vi "hmi_simRK4serial.vi"() -> ()   [LabVIEW 2017]
uses:
  Control 6.ctl
  <vilib>/Utility/miscctls.llb/LVBoundsTypeDef.ctl
  <vilib>/Instr/_visa.llb/VISA Configure Serial Port (Instr).vi
  <vilib>/MakerHub/LINX/LMH-LINX.lvlib
panel:
  in  "ENVIAR":bool=TRUE
  out "bomba":dbl
  out "dato a enviar":string
  in  "stop":bool
  out "time array":dbl[](array[numeric])
  in  "Tab Control":enum32{"HMI", "Monitorizacion de flujo"}(tab)
  out "Boolean 2":bool
  out "FUGA 1":bool
  out "FUGA 2":bool
  out "u2":dbl=3.4 format="%#_13g"
  out "Boolean":bool
  in  "BOMBA ON/OFF":bool
  out "FT1":bool(c317)
  in  "valvula 1":bool
  in  "valvula 2":bool
  out "TEE 02":bool
  out "TUBERIA 1IN TRAMO 02":bool(c317)
  out "TEE1":bool
  out "Multi-Segment Pipe 2":T1
  out "Multi-Segment Pipe 3":bool(c317)
  out "Multi-Segment Pipe 4":bool(c317)
  out "FT2":bool(c317)
  out "FT 1":dbl caption="L/min"
  out "FT 2":dbl caption="L/min"
  out "67.5°":bool
  out "45°":bool
  out "22.5°":bool
  out "90°":bool
  out "TANQUE\n FLUIDO:AGUA":dbl(slide) scale=0.0..100.0
  out "SENSOR FLUJO":bool
  out "67.5° 3":bool
  out "45° 3":bool
  out "22.5° 3":bool
  out "90° 3":bool
  out "SENSOR FLUJO 3":bool
  out "BOMBA 1/2 HP":bool
  out "tiempo":dbl
  in  "Flujo de entrada":dbl=0.00425 format="%#_13g"
  out "codo90":bool
  out "u1":dbl=6.0 format="%#_13g"
  in  "Tiempo muestreo":i32=200
  out "periodo":dbl
  in  "Flujo de salida":dbl=0.00425 format="%#_13g"
  out "element":dbl
  out "element 2":dbl
  in  "Puerto sensores":refnum<visa-resource-name>="COM3"
  in  "GUARDAR DATOS":bool
  out "Flujo de entrada y salida":cluster{dbl[], dbl[]}[](graph)
  out "Freq2":dbl
  out "Freq1":dbl
  out "Cluster":T2
  out "SIMULACION DE Q1 y Q2":cluster{dbl[], dbl[]}[](graph)
  out "SIMULACION DE H2":cluster{"time array":dbl[], dbl[]}(graph)
  # "PVC  1\" FLUJO: AGUA"
  # "PVC  1/2\" FLUJO: AGUA"
  # "FUGA 1"
  # "2.5 m"
  # "PVC  1/2\" FLUJO: AGUA"
  # "FUGA 2"
  # "PVC  1\" FLUJO: AGUA"
  # "6 m"
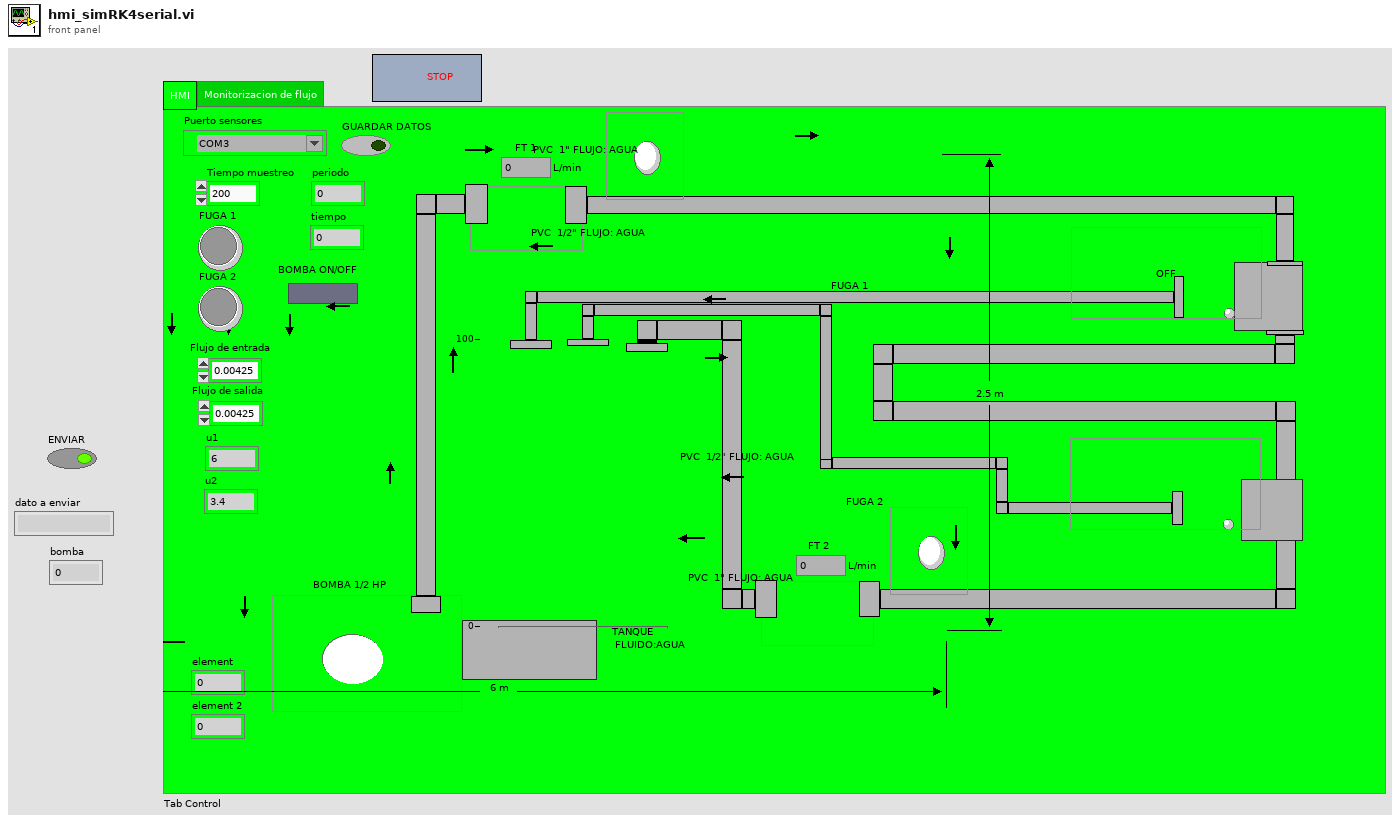
[diagram p1: front panel]
types:
  T1 = typedef "Control 6.ctl" = bool
  T2 = cluster{"FLUJO DE ENTRADA":dbl, "FLUJO DE SALIDA":dbl, "VOLUMEN 1 (L) ":dbl, "VOLUMEN 2 (L) ":dbl}
  T3 = typedef "LVBoundsTypeDef.ctl" = cluster{"Width":u32, "Height":u32}
  T4 = cluster{"index":i32, "index 2":i32, "index 3":i32, "index 4":i32, "index 5":i32, "index 6":i32, i32, i32, i32}
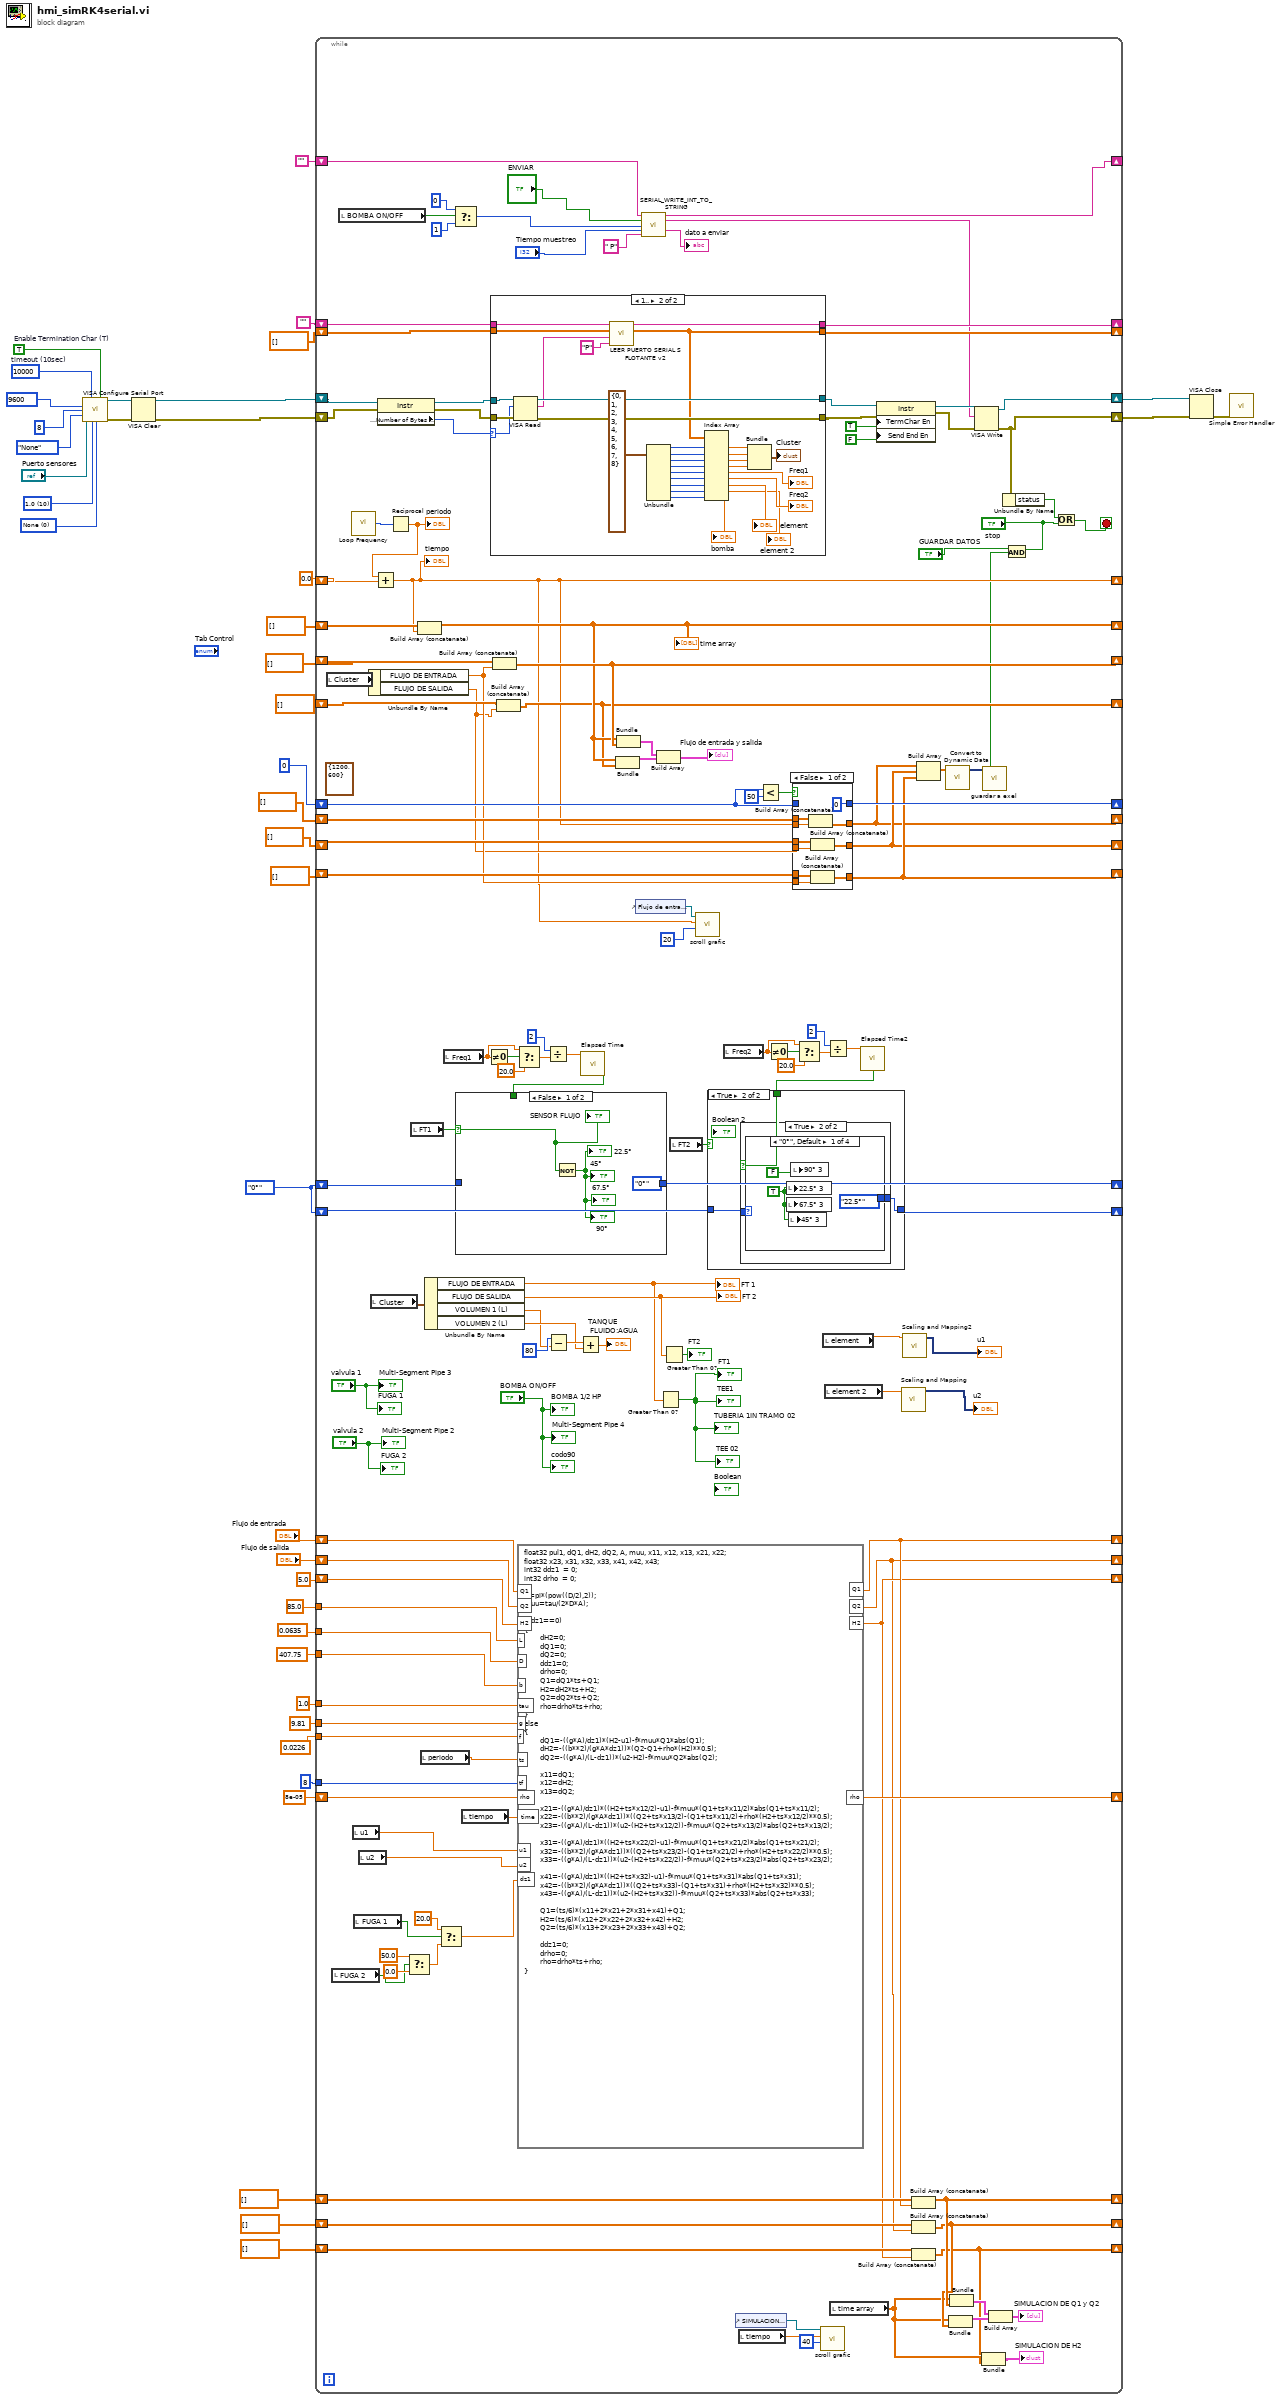
[diagram p0: block diagram]
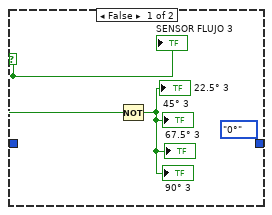
[diagram p2: hidden frame]
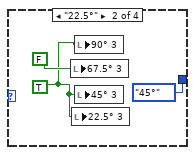
[diagram p4: hidden frame]
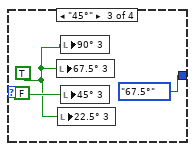
[diagram p5: hidden frame]
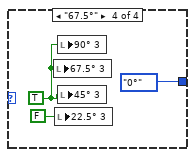
[diagram p6: hidden frame]
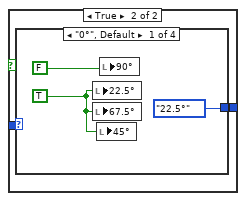
[diagram p8: hidden frame]
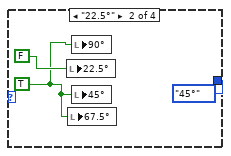
[diagram p9: hidden frame]
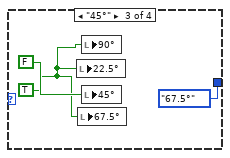
[diagram p10: hidden frame]
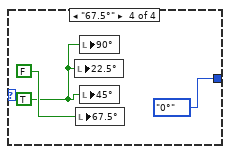
[diagram p11: hidden frame]
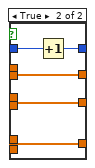
[diagram p12: hidden frame]
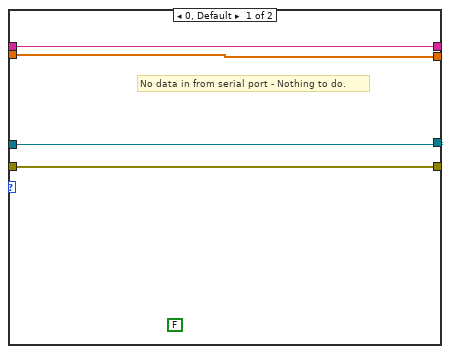
[diagram p13: hidden frame]
diagram:
  w21 = 9600 items=["9600"=9600, "19200"=19200, "38400"=38400, "57600"=57600, "74880"=74880, "115200"=115200] ("BaudRate")
  w20 = enum16{"0°", "22.5°", "45°", "67.5°"}."0°"
  w33 = u16 10 items=["1.0"=10, "1.5"=15, "2.0"=20] ("stop bits (10: 1 bit)")
  w34 = u16 0 items=["None", "XON/XOFF", "RTS/CTS", "XON/XOFF & RTS/CTS", "DTR/DSR", "XON/XOFF & DTR/DSR"] ("flow control (0:none)")
  w39 = TRUE  # Enable Termination Char (T)
  w40 = u32 10000  # timeout (10sec)
  (unwired) T3 {"Width"=1200, "Height"=600} ("Tab Control Pane Dimension")
  n1 = call-poly "VISA Configure Serial Port"("VISA resource name"="Puerto sensores", "timeout (10sec)"=w40, "Enable Termination\nChar (T)"=w39, "baud rate (9600)"=w21, "data bits (8)"=u16 8 ("Data bits (8)"), "parity (0:none)"=enum16{"None", "Odd", "Even", "Mark", "Space"}."None" ("Parity (0:none)"), "stop bits (10: 1 bit)"=w33, "flow control (0:none)"=w34) -> ("VISA resource name out"=w37:refnum<visa-resource-name>, "error out"=w38:errorcluster)  [unwired: 6 in]
  n2 = VISA Clear(VISA resource name=w37, error in (no error)=w38) -> (VISA resource name out=w36:refnum<visa-resource-name>, error out=w2:errorcluster)
  n3 = while {
    shift-right: [w155] -> _
    shift-left: dbl[] [] -> [w175]
    shift-right: [w72] -> _
    shift-left: 0.0 -> [w176]
    shift-right: [w168] -> _
    shift-left: dbl[] [] -> [w173]
    shift-right: [w154] -> _
    shift-left: dbl[] [] -> [w174]
    shift-right: [w165] -> _
    shift-left: 0 -> [w166]
    shift-right: [w160] -> _
    shift-left: dbl[] [] -> [w163]
    shift-right: [w161] -> _
    shift-left: dbl[] [] -> [w162]
    shift-right: [w159] -> _
    shift-left: dbl[] [] -> [w164]
    shift-right: [w58] -> w41
    shift-left: w2 -> [w60]
    shift-right: [w45] -> w22
    shift-left: w36 -> [w179]
    shift-right: [w140] -> _
    shift-left: w20 -> [w139]
    shift-right: [w120] -> _
    shift-left: w20 -> [w129]
    shift-right: [w116] -> _
    shift-left: "" -> [w117]
    shift-right: [w114] -> _
    shift-left: dbl[] [] -> [w115]
    tunnel: 0.0226 ("input variable") -> [w112]
    tunnel: 9.81 ("input variable") -> [w111]
    tunnel: 1.0 ("input variable") -> [w110]
    tunnel: 407.75 ("input variable") -> [w109]
    tunnel: 0.0635 ("D") -> [w108]
    tunnel: 85.0 ("L") -> [w107]
    shift-right: [w87] -> _
    shift-left: "Flujo de entrada" -> [w106]
    shift-right: [w76] -> _
    shift-left: "Flujo de salida" -> [w105]
    shift-right: [w84] -> _
    shift-left: 5.0 -> [w104]
    shift-right: [w102] -> _
    shift-left: 8e-05 -> [w103]
    tunnel: 8 -> [w101]
    shift-right: [w80] -> _
    shift-left: dbl[] [] -> [w88]
    shift-right: [w79] -> _
    shift-left: dbl[] [] -> [w86]
    shift-right: [w68] -> _
    shift-left: dbl[] [] -> [w85]
    shift-right: [w55] -> _
    shift-left: "" -> [w56]
    stop <- w113 stop-if-true
    n4 = local read "Cluster"() -> (w153:T2)
    n5 = local read "FUGA 2"() -> (w94:bool)
    n6 = local read "BOMBA ON/OFF"() -> (w50:bool)
    n7 = call <vilib>:"Loop Frequency.vi"() -> ("Loop Rate (Hz)"=w170:u32)
    n8 = local read "u1"() -> (w74:dbl)
    n9 = local read "FUGA 1"() -> (w95:bool)
    n10 = local read "u2"() -> (w73:dbl)
    n11 = Unbundle By Name(w153) -> ("FLUJO DE ENTRADA"=w152:dbl, "FLUJO DE SALIDA"=w151:dbl)
    n12 = local read "Cluster"() -> (w143:T2)
    n13 = property class="Instr"(reference=w179, error in=w60) -> (reference out=w181:refnum<visa-resource-name>, error out=w180:errorcluster, "Serial Settings:Number of Bytes at Serial Port"=w178:u32)
    n14 = Reciprocal(x=w170) -> (1/x=w172:dbl)
    "periodo" <- w172
    n15 = Add(x=w172, y=w176) -> (x+y=w72:dbl)
    "tiempo" <- w72
    n16 = Select(t=50.0, s=w94, f=0.0) -> (s? t:f=w99:dbl)
    n17 = local read "FT1"() -> (w141:bool)
    n18 = Build Array (concatenate)(w175, w72) -> (w155:dbl[])
    "time array" <- w155
    n19 = local read "periodo"() -> (w75:dbl)
    n20 = Unbundle By Name(w143) -> ("FLUJO DE ENTRADA"=w142:dbl, "FLUJO DE SALIDA"=w149:dbl, "VOLUMEN 1 (L)"=w118:dbl, "VOLUMEN 2 (L)"=w144:dbl)
    "FT 1" <- w142
    "FT 2" <- w149
    n21 = Select(t=20.0, s=w95, f=w99) -> (s? t:f=w96:dbl)
    n22 = local read "Freq1"() -> (w137:dbl)
    n23 = Select(t=0, s=w50, f=1) -> (s? t:f=w47:i32)
    n24 = local read "tiempo"() -> (w93:dbl)
    n25 = Not Equal To 0?(x=w137) -> (x != 0?=w138:bool)
    n26 = case shown="1.." w178 {
      selector: w178 -> [_ w269]
      tunnel: [w241 w273] -> w59
      tunnel: [w242 w272] -> w46
      tunnel: w181 -> [w242 w271]
      tunnel: w180 -> [w241 w270]
      tunnel: w117 -> [w240 w259]
      tunnel: [w240 w258] -> w116
      tunnel: w115 -> [w239 w257]
      tunnel: [w239 w256] -> w114
      frame 0, Default {
        (unwired) FALSE
        # "No data in from serial port - Nothing to do."
      }
      frame 1.. {
        n27 = VISA Read(VISA resource name=w271, byte count=w269, error in (no error)=w270) -> (VISA resource name out=w272:refnum<visa-resource-name>, read buffer=w260:string, error out=w273:errorcluster)  [unwired: 1 out]
        n28 = call <userlib>:"LEER PUERTO SERIAL S FLOTANTE v2.vi"("caracter terminador"="P" ("regular expression"), "read buffer"=w260, "buffer de datos"=w257, "buffer in"=w259) -> ("salida datos numericos"=w256:dbl[], "buffer out"=w258:string)  [unwired: 1 in, 1 out]
        n29 = Unbundle(T4 {"index"=0, "index 2"=1, "index 3"=2, "index 4"=3, "index 5"=4, "index 6"=5, 6, 7, 8}) -> ("index"=w254:i32, "index 2"=w253:i32, "index 3"=w252:i32, "index 4"=w251:i32, "index 5"=w250:i32, "index 6"=w249:i32, w248:i32, w247:i32, w244:i32)
        n30 = Index Array(array=w256, index #1=w254, index #2=w253, index #3=w252, index #4=w251, index #5=w250, index #6=w249, index #7=w248, index #8=w247, index #9=w244) -> (element #1=w267:dbl, element #2=w266:dbl, element #3=w264:dbl, element #4=w265:dbl, element #5=→"Freq1":dbl, element #6=→"Freq2":dbl, element #7=→"element":dbl, element #8=→"element 2":dbl, element #9=→"bomba":dbl)
        n31 = Bundle(w267, w266, w264, w265) -> (→"Cluster":cluster{dbl, dbl, dbl, dbl})  [unwired: 1 in]
      }
    }
    n32 = Build Array (concatenate)(w173, w152) -> (w168:dbl[])
    n33 = Build Array (concatenate)(w174, w151) -> (w154:dbl[])
    n34 = Select(t=w137, s=w138, f=20.0) -> (s? t:f=w135:dbl)
    n35 = formula code="float32 pul1, dQ1, dH2, dQ2, A, muu, x11, x12, x13, x21, x22;\nfloat32 x23, x31, x32, x33, x41, x42, x43;\nint32 ddz1  = 0;\nint32 drho  = 0;\n\nA=pi*(pow((D/2),2));\nmuu=tau/(2*D*A);\n\nif(dz1==0)\n{\n        dH2=0;\n        dQ1=0;\n        dQ2=0;\n        ddz1=0;\n        drho=0;\n        Q1=dQ1*ts+Q1;\n        H2=dH2*ts+H2;    \n        Q2=dQ2*ts+Q2;\n        rho=drho*ts+rho;\n}\nelse \n{\n        dQ1=-((g*A)/dz1)*(H2-u1)-f*muu*Q1*abs(Q1);\n        dH2=-((b**2)/(g*A*dz1))*(Q2-Q1+rho*(H2)**0.5);\n        dQ2=-((g*A)/(L-dz1))*(u2-H2)-f*muu*Q2*abs(Q2);\n        \n        x11=dQ1;\n        x12=dH2;\n        x13=dQ2;\n        \n        x21=-((g*A)/dz1)*((H2+ts*x12/2)-u1)-f*muu*(Q1+ts*x11/2)*abs(Q1+ts*x11/2);\n        x22=-((b**2)/(g*A*dz1))*((Q2+ts*x13/2)-(Q1+ts*x11/2)+rho*(H2+ts*x12/2)**0.5);\n        x23=-((g*A)/(L-dz1))*(u2-(H2+ts*x12/2))-f*muu*(Q2+ts*x13/2)*abs(Q2+ts*x13/2);\n        \n        x31=-((g*A)/dz1)*((H2+ts*x22/2)-u1)-f*muu*(Q1+ts*x21/2)*abs(Q1+ts*x21/2);\n        x32=-((b**2)/(g*A*dz1))*((Q2+ts*x23/2)-(Q1+ts*x21/2)+rho*(H2+ts*x22/2)**0.5);\n        x33=-((g*A)/(L-dz1))*(u2-(H2+ts*x22/2))-f*muu*(Q2+ts*x23/2)*abs(Q2+ts*x23/2);\n        \n        x41=-((g*A)/dz1)*((H2+ts*x32)-u1)-f*muu*(Q1+ts*x31)*abs(Q1+ts*x31);\n        x42=-((b**2)/(g*A*dz1))*((Q2+ts*x33)-(Q1+ts*x31)+rho*(H2+ts*x32)**0.5);\n        x43=-((g*A)/(L-dz1))*(u2-(H2+ts*x32))-f*muu*(Q2+ts*x33)*abs(Q2+ts*x33);\n        \n        Q1=(ts/6)*(x11+2*x21+2*x31+x41)+Q1;\n        H2=(ts/6)*(x12+2*x22+2*x32+x42)+H2;\n        Q2=(ts/6)*(x13+2*x23+2*x33+x43)+Q2;\n        \n        ddz1=0;\n        drho=0;\n        rho=drho*ts+rho;\n}"("L"=w107, "D"=w108, "b"=w109, "tau"=w110, "g"=w111, "Q1"=w106, "Q2"=w105, "f"=w112, "ts"=w75, "tf"=w101, "rho"=w103, "H2"=w104, "time"=w93, "u1"=w74, "u2"=w73, "dz1"=w96) -> ("rho"=w102:dbl, "Q1"=w87:dbl, "Q2"=w76:dbl, "H2"=w84:dbl)
    n36 = Divide(x=i8 2, y=w135) -> (x/y=w134:dbl)
    n37 = Subtract(x=80, y=w118) -> (x-y=w145:dbl)
    n38 = Add(x=w145, y=w144) -> (x+y=→"TANQUE\n FLUIDO:AGUA":dbl)
    n39 = call "Elapsed Time"("Time Target (s)"=w134) -> ("Time has Elapsed"=w132:bool)  [unwired: 11 in, 7 out]
    n40 = case shown="False" w141 {
      selector: w141 -> [w205 _]
      tunnel: w139 -> [_ w208]
      tunnel: [enum16{"0°", "22.5°", "45°", "67.5°"}."0°" w207] -> w140
      tunnel: w132 -> [_ w206]
      frame False {
        n41 = Not(x=w205) -> (.not. x?=→"90°" →"22.5°" →"45°" →"67.5°":bool)
        "SENSOR FLUJO" <- w205
      }
      frame True {
        n42 = case shown="False" w206 {
          tunnel: w208 -> [w209 w211]
          tunnel: [w209 w210] -> w207
          frame False {
          }
          frame True {
            n43 = case shown="\"0°\", Default" w211 {
              tunnel: [enum16{"0°", "22.5°", "45°", "67.5°"}."22.5°" enum16{"0°", "22.5°", "45°", "67.5°"}."45°" enum16{"0°", "22.5°", "45°", "67.5°"}."67.5°" enum16{"0°", "22.5°", "45°", "67.5°"}."0°"] -> w210
              frame "0°", Default {
                w212 = TRUE
                n44 = local write "22.5°"(w212) -> ()
                n45 = local write "67.5°"(w212) -> ()
                n46 = local write "45°"(w212) -> ()
                n47 = local write "90°"(FALSE) -> ()
              }
              frame "22.5°" {
                w215 = TRUE
                n48 = local write "22.5°"(FALSE) -> ()
                n49 = local write "67.5°"(w215) -> ()
                n50 = local write "90°"(w215) -> ()
                n51 = local write "45°"(w215) -> ()
              }
              frame "45°" {
                w218 = TRUE
                n52 = local write "22.5°"(w218) -> ()
                n53 = local write "67.5°"(w218) -> ()
                n54 = local write "90°"(w218) -> ()
                n55 = local write "45°"(FALSE) -> ()
              }
              frame "67.5°" {
                w221 = TRUE
                n56 = local write "22.5°"(w221) -> ()
                n57 = local write "67.5°"(FALSE) -> ()
                n58 = local write "90°"(w221) -> ()
                n59 = local write "45°"(w221) -> ()
              }
            }
          }
        }
      }
    }
    n60 = Bundle(w155, w154) -> (w78:cluster{dbl[], dbl[]})  [unwired: 1 in]
    n61 = Bundle(w155, w168) -> (w171:cluster{dbl[], dbl[]})  [unwired: 1 in]
    n62 = control-ref of="Flujo de entrada y salida"() -> (w83:refnum<vi>)
    n63 = call <userlib>:"SERIAL_WRITE_INT_TO_STRING.vi"("buffer in"=w56, "ENVIAR"="ENVIAR", "bomba on/off"=w47, "tiempo"="Tiempo muestreo", "fin de cadena"=" P") -> ("buffer out"=w55:string, "int to string out"=w54:string, "dato a enviar"=→"dato a enviar":string)  [unwired: 7 in, 1 out]
    n64 = Build Array(w171, w78) -> (→"Flujo de entrada y salida":cluster{dbl[], dbl[]}[])
    n65 = Greater Than 0?(x=w142) -> (x > 0?=→"TUBERIA 1IN TRAMO 02" →"TEE1" →"TEE 02" →"FT1":bool)
    n66 = Greater Than 0?(x=w149) -> (x > 0?=→"FT2":bool)
    n67 = local read "FT2"() -> (w121:bool)
    n68 = call <userlib>:"scroll grafic.vi"("Rango de grafica"=i16 20, "tiempo"=w72, "XYGraph in"=w83) -> ()  [unwired: 9 in]
    n69 = local read "Freq2"() -> (w127:dbl)
    n70 = control-ref of="SIMULACION DE Q1 y Q2"() -> (w67:refnum<vi>)
    n71 = local read "tiempo"() -> (w65:dbl)
    n72 = Less?(x=w166, y=u32 50) -> (x < y?=w156:bool)
    n73 = Not Equal To 0?(x=w127) -> (x != 0?=w128:bool)
    n74 = case shown="False" w156 {
      tunnel: w166 -> [_ w238]
      tunnel: [u32 0 w237] -> w165
      tunnel: w164 -> [w232 w234]
      tunnel: w151 -> [w230 _]
      tunnel: [w233 w236] -> w160
      tunnel: w163 -> [w231 w236]
      tunnel: w152 -> [w228 _]
      tunnel: w162 -> [w229 w235]
      tunnel: [w227 w235] -> w161
      tunnel: [w226 w234] -> w159
      tunnel: w72 -> [w225 _]
      frame False {
        n75 = Build Array (concatenate)(w232, w225) -> (w226:dbl[])
        n76 = Build Array (concatenate)(w231, w230) -> (w233:dbl[])
        n77 = Build Array (concatenate)(w229, w228) -> (w227:dbl[])
      }
      frame True {
        n78 = Increment(x=w238) -> (x+1=w237:u32)
      }
    }
    n79 = Select(t=w127, s=w128, f=20.0) -> (s? t:f=w125:dbl)
    n80 = call <userlib>:"scroll grafic.vi"("Rango de grafica"=i16 40, "tiempo"=w65, "XYGraph in"=w67) -> ()  [unwired: 9 in]
    n81 = local read "element"() -> (w90:dbl)
    n82 = local read "element 2"() -> (w89:dbl)
    n83 = Divide(x=i8 2, y=w125) -> (x/y=w124:dbl)
    n84 = local read "time array"() -> (w69:dbl[])
    n85 = call "Elapsed Time2"("Time Target (s)"=w124) -> ("Time has Elapsed"=w122:bool)  [unwired: 11 in, 7 out]
    n86 = case shown="True" w121 {
      selector: w121 -> [w184 _]
      tunnel: w129 -> [_ w187]
      tunnel: [enum16{"0°", "22.5°", "45°", "67.5°"}."0°" w186] -> w120
      tunnel: w122 -> [_ w185]
      frame False {
        n87 = Not(x=w184) -> (.not. x?=→"90° 3" →"22.5° 3" →"45° 3" →"67.5° 3":bool)
        "SENSOR FLUJO 3" <- w184
      }
      frame True {
        n88 = case shown="True" w185 {
          tunnel: w187 -> [w188 w190]
          tunnel: [w188 w189] -> w186
          frame False {
          }
          frame True {
            n89 = case shown="\"0°\", Default" w190 {
              tunnel: [enum16{"0°", "22.5°", "45°", "67.5°"}."22.5°" enum16{"0°", "22.5°", "45°", "67.5°"}."45°" enum16{"0°", "22.5°", "45°", "67.5°"}."67.5°" enum16{"0°", "22.5°", "45°", "67.5°"}."0°"] -> w189
              frame "0°", Default {
                w191 = TRUE
                n90 = local write "22.5° 3"(w191) -> ()
                n91 = local write "67.5° 3"(w191) -> ()
                n92 = local write "45° 3"(w191) -> ()
                n93 = local write "90° 3"(FALSE) -> ()
              }
              frame "22.5°" {
                w194 = TRUE
                n94 = local write "67.5° 3"(FALSE) -> ()
                n95 = local write "22.5° 3"(w194) -> ()
                n96 = local write "90° 3"(w194) -> ()
                n97 = local write "45° 3"(w194) -> ()
              }
              frame "45°" {
                w197 = TRUE
                n98 = local write "67.5° 3"(w197) -> ()
                n99 = local write "22.5° 3"(w197) -> ()
                n100 = local write "90° 3"(w197) -> ()
                n101 = local write "45° 3"(FALSE) -> ()
              }
              frame "67.5°" {
                w200 = TRUE
                n102 = local write "67.5° 3"(w200) -> ()
                n103 = local write "22.5° 3"(FALSE) -> ()
                n104 = local write "90° 3"(w200) -> ()
                n105 = local write "45° 3"(w200) -> ()
              }
            }
          }
        }
      }
    }
    n106 = property class="Instr"(reference=w46, error in=w59, "TermChar En"=TRUE ("Message Based Settings:Termination Character Enable"), "Send End En"=FALSE ("Message Based Settings:Send End Enable")) -> (reference out=w62:refnum<visa-resource-name>, error out=w61:errorcluster)
    n107 = call "Scaling and Mapping"("Signals"=w89) -> ("Scaled Signals"=→"u2":dynamicdata)  [unwired: 9 in, 1 out]
    n108 = call "Scaling and Mapping2"("Signals"=w90) -> ("Scaled Signals"=→"u1":dynamicdata)  [unwired: 9 in, 1 out]
    n109 = Build Array (concatenate)(w88, w87) -> (w80:dbl[])
    n110 = Build Array (concatenate)(w86, w76) -> (w79:dbl[])
    n111 = Build Array (concatenate)(w85, w84) -> (w68:dbl[])
    n112 = Build Array(w159, w160, w161) -> (w157:dbl[][])
    n113 = call "Convert to Dynamic Data"("2D Array"=w157) -> ("Dynamic Data Type"=w158:dynamicdata)  [unwired: 3 in]
    n114 = Bundle("time array"=w69, w79) -> (w81:cluster{"time array":dbl[], dbl[]})  [unwired: 1 in]
    n115 = Bundle("time array"=w69, w80) -> (w82:cluster{"time array":dbl[], dbl[]})  [unwired: 1 in]
    n116 = VISA Write(VISA resource name=w62, write buffer=w54, error in (no error)=w61) -> (VISA resource name out=w45:refnum<visa-resource-name>, error out=w58:errorcluster)  [unwired: 1 out]
    n117 = Bundle("time array"=w69, w68) -> (→"SIMULACION DE H2":cluster{"time array":dbl[], dbl[]})  [unwired: 1 in]
    n118 = Build Array(w82, w81) -> (→"SIMULACION DE Q1 y Q2":cluster{"time array":dbl[], dbl[]}[])
    n119 = Unbundle By Name(w58) -> ("status"=w177:bool)
    n120 = And(x="stop", y="GUARDAR DATOS") -> (x .and. y?=w53:bool)
    n121 = call "guardar a exel"("Signals"=w158, "Enable"=w53) -> ()  [unwired: 15 in, 3 out]
    n122 = Or(x=w177, y="stop") -> (x .or. y?=w113:bool)
    "BOMBA 1/2 HP" <- "BOMBA ON/OFF"
    "codo90" <- "BOMBA ON/OFF"
    "Multi-Segment Pipe 4" <- "BOMBA ON/OFF"
    "Multi-Segment Pipe 3" <- "valvula 1"
    "Multi-Segment Pipe 2" <- "valvula 2"
    "FUGA 2" <- "valvula 2"
    "FUGA 1" <- "valvula 1"
  }
  n123 = VISA Close(VISA resource name=w22, error in (no error)=w41) -> (error out=w1:errorcluster)
  n124 = call <vilib>:"Simple Error Handler.vi"("error in (no error)"=w1) -> ()  [unwired: 4 in, 5 out]
